vi "Wait.vi"(0 "Parallel Task in":refnum<k21>, 1 "PS type":enum16{"NHR", "ITECH"}(ring), 5 "P task error in":errorcluster, 9 "PS VISA in":refnum<visa-resource-name>, 11 "PS error in":errorcluster caption="NHR error in (no error)", 12 "Wait Filepath":path=path "C:/Users/ga11/Desktop/VI/results/3PtestChrgRest.lvm" caption="Filename", 13 "Wait time":dbl) -> (4 "parallel task out":refnum<k21>, 6 "parallel task error out":errorcluster, 10 "PS Visa Out":refnum<visa-resource-name>, 15 "PS error out":errorcluster)   [LabVIEW 2020]
uses:
  <instrlib>/NH Research Regenerative Test Series/Public/Data/Read (Ave Current).vi
  <instrlib>/NH Research Regenerative Test Series/Public/Data/Low Level/Fetch (Ave Voltage).vi
  <instrlib>/NH Research Regenerative Test Series/NH Research Regenerative Test Series.lvlib
  <instrlib>/IT-M3400/IT-M3400.lvlib
panel:
  out "Ave Current (A)":dbl
  out "Ave Voltage (V)":dbl
  out "WaitElapsed Time (s)":i32 caption="Elapsed Time (s)"
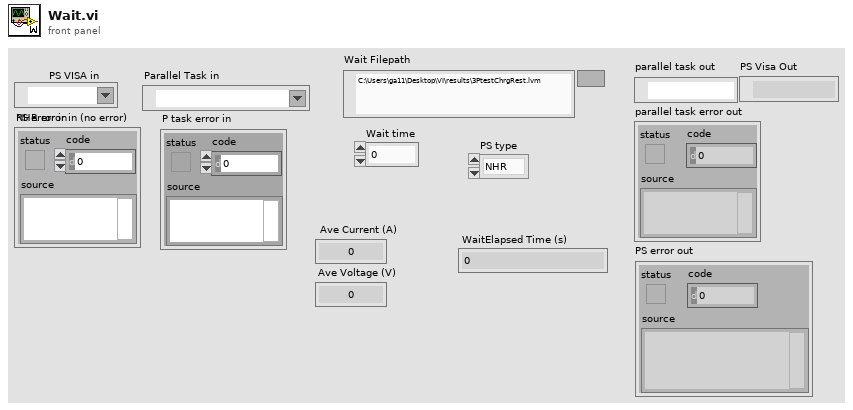
[diagram p1: front panel]
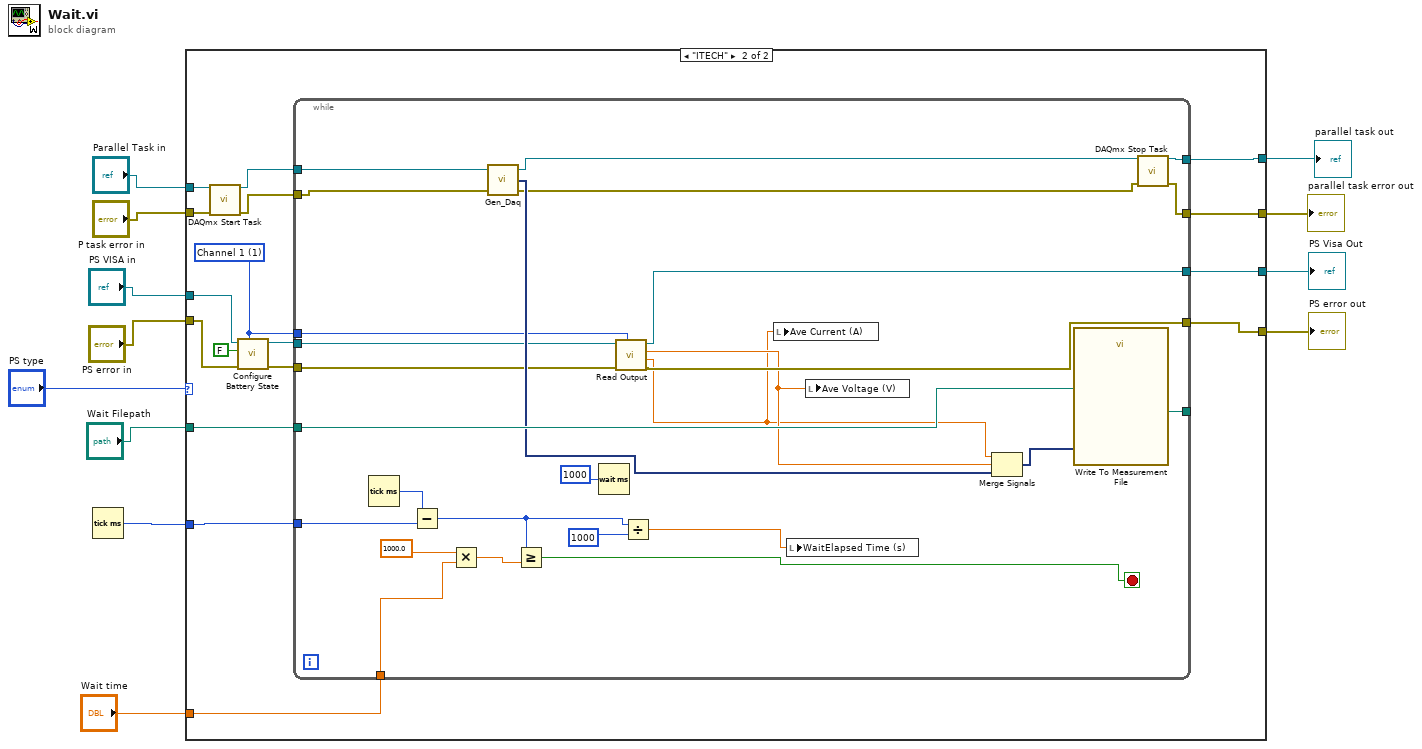
[diagram p0: block diagram]
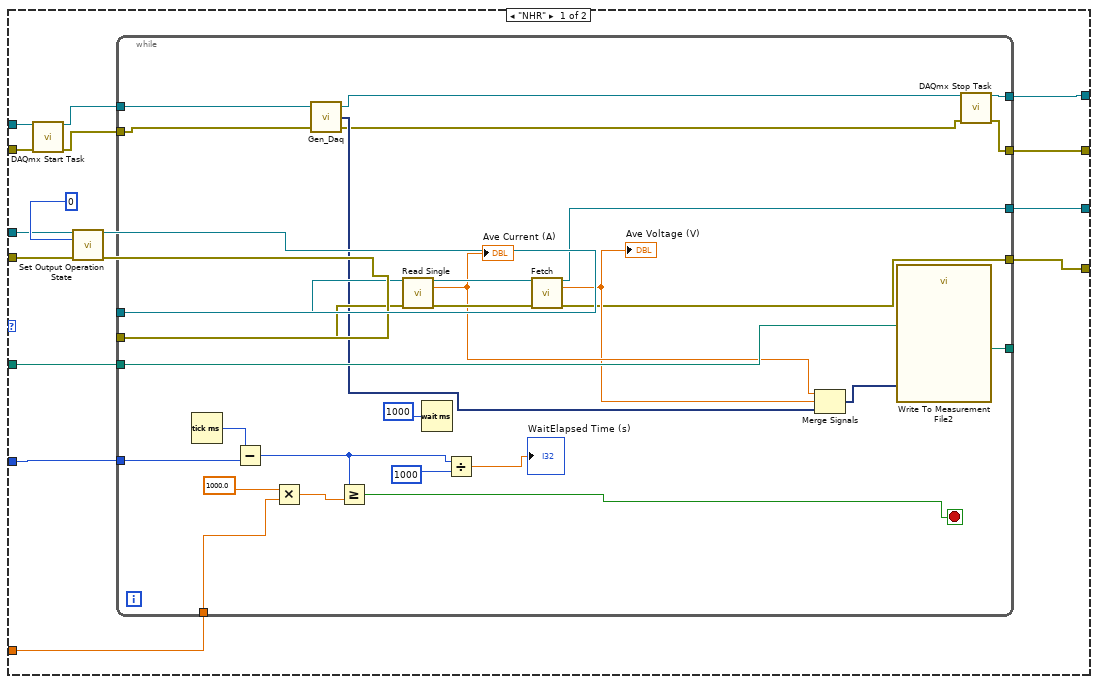
[diagram p2: hidden frame]
diagram:
  n1 = Tick Count (ms)() -> (millisecond timer value=w11:u32)
  n2 = case shown="\"ITECH\"" "PS type" {
    tunnel: "Wait time" -> [w25 w73]
    tunnel: w11 -> [w22 w70]
    tunnel: "Parallel Task in" -> [w21 w69]
    tunnel: "P task error in" -> [w20 w68]
    tunnel: "PS VISA in" -> [w19 w60]
    tunnel: "PS error in" -> [w18 w59]
    tunnel: "Wait Filepath" -> [w17 w67]
    tunnel: [w16 w66] -> w5
    tunnel: [w15 w65] -> w4
    tunnel: [w14 w64] -> w3
    tunnel: [w13 w63] -> w2
    frame "NHR" {
      n3 = call <vilib>:"DAQmx Start Task.vi"("task/channels in"=w21, "error in"=w20) -> ("task out"=w24:refnum<k21>, "error out"=w23:errorcluster)  [unwired: 12 in]
      n4 = call <vilib>:"Set Output Operation State.vi"("VISA resource name"=w19, "Mode (0: Off)"=0, "error in (no error)"=w18) -> ("VISA resource name out"=w27:refnum<visa-resource-name>, "error out"=w26:errorcluster)  [unwired: 11 in]
      n5 = while {
        tunnel: w27 -> [w54]
        tunnel: w26 -> [w53]
        tunnel: w25 -> [w49]
        tunnel: [w46] -> _
        tunnel: w24 -> [w36]
        tunnel: w23 -> [w35]
        tunnel: w22 -> [w45]
        tunnel: w17 -> [w44]
        tunnel: [w43] -> w16
        tunnel: [w42] -> w15
        tunnel: [w33] -> w14
        tunnel: [w32] -> w13
        stop <- w50 stop-if-true
        n6 = Tick Count (ms)() -> (millisecond timer value=w51:u32)
        n7 = Subtract(x=w51, y=w45) -> (x-y=w41:u32)
        n8 = Multiply(x=1000.0, y=w49) -> (x*y=w47:dbl)
        n9 = call "Gen_Daq.vi"("error in"=w35, "task/channels in"=w36) -> ("error out"=w29:errorcluster, "DaQ_output"=w31:dynamicdata, "task out"=w30:refnum<k21>)  [unwired: 1 in]
        n10 = Greater Or Equal?(x=w41, y=w47) -> (x >= y?=w50:bool)
        n11 = call-poly <instrlib>:"Read Single.vi"("VISA resource name"=w54, "error in (no error)"=w53) -> ("VISA resource name out"=w55:refnum<visa-resource-name>, "Ave Current (A)"=w38:dbl, "error out"=w56:errorcluster)  [unwired: 11 in]
        "Ave Current (A)" <- w38
        n12 = Wait (ms)(milliseconds to wait=1000) -> ()  [unwired: 1 out]
        n13 = Divide(x=w41, y=1000) -> (x/y=→"WaitElapsed Time (s)":dbl)
        n14 = call-poly <instrlib>:"Fetch.vi"("VISA resource name"=w55, "error in (no error)"=w56) -> ("VISA resource name out"=w33:refnum<visa-resource-name>, "Ave Voltage (V)"=w34:dbl, "error out"=w32:errorcluster)  [unwired: 11 in]
        "Ave Voltage (V)" <- w34
        n15 = Merge Signals "Merge Signals"(w38, w34, w31) -> (w37:dynamicdata)
        n16 = call "Write To Measurement File2"("Signals"=w37, "Filename"=w44) -> ("Filename Out"=w46:path)  [unwired: 15 in, 2 out]
        n17 = call <vilib>:"DAQmx Stop Task.vi"("task/channels in"=w30, "error in"=w29) -> ("task out"=w43:refnum<k21>, "error out"=w42:errorcluster)  [unwired: 12 in]
      }
    }
    frame "ITECH" {
      w57 = 1 items=["Channel 1"=1, "Channel 2"=2, "Channel 3"=3, "Channel 4"=4, "Channel 5"=5, "Channel 6"=6, "Channel 7"=7, "Channel 8"=8, "Channel 8"=9, "Channel 10"=10, "Channel 11"=11, "Channel 12"=12, "Channel 13"=13, "Channel 14"=14, "Channel 15"=15, "Channel 16"=16] ("Channel")
      n18 = call <vilib>:"DAQmx Start Task.vi"("task/channels in"=w69, "error in"=w68) -> ("task out"=w72:refnum<k21>, "error out"=w71:errorcluster)  [unwired: 12 in]
      n19 = call <instrlib>:"Configure Battery State.vi"("Channel"=w57, "error in"=w59, "State"=FALSE, "VISA resource name"=w60) -> ("error out"=w61:errorcluster, "VISA resource name out"=w62:refnum<visa-resource-name>)  [unwired: 6 in]
      n20 = while {
        tunnel: w73 -> [w97]
        tunnel: [w94] -> _
        tunnel: w72 -> [w86]
        tunnel: w71 -> [w85]
        tunnel: w70 -> [w93]
        tunnel: w67 -> [w92]
        tunnel: [w91] -> w66
        tunnel: [w90] -> w65
        tunnel: [w81] -> w64
        tunnel: [w80] -> w63
        tunnel: w62 -> [w76]
        tunnel: w61 -> [w75]
        tunnel: w57 -> [w74]
        stop <- w98 stop-if-true
        n21 = Tick Count (ms)() -> (millisecond timer value=w99:u32)
        n22 = Subtract(x=w99, y=w93) -> (x-y=w89:u32)
        n23 = Multiply(x=1000.0, y=w97) -> (x*y=w95:dbl)
        n24 = call "Gen_Daq.vi"("error in"=w85, "task/channels in"=w86) -> ("error out"=w82:errorcluster, "DaQ_output"=w84:dynamicdata, "task out"=w83:refnum<k21>)  [unwired: 1 in]
        n25 = Greater Or Equal?(x=w89, y=w95) -> (x >= y?=w98:bool)
        n26 = Wait (ms)(milliseconds to wait=1000) -> ()  [unwired: 1 out]
        n27 = call <instrlib>:"Read Output.vi"("Channel"=w74, "error in"=w75, "VISA resource name"=w76) -> ("error out"=w80:errorcluster, "Read Current(A)"=w78:dbl, "Read Voltage(V)"=w79:dbl, "VISA resource name out"=w81:refnum<visa-resource-name>)  [unwired: 5 in]
        n28 = Divide(x=w89, y=1000) -> (x/y=w77:dbl)
        n29 = local write "Ave Current (A)"(w78) -> ()
        n30 = local write "WaitElapsed Time (s)"(w77) -> ()
        n31 = local write "Ave Voltage (V)"(w79) -> ()
        n32 = Merge Signals "Merge Signals"(w78, w79, w84) -> (w87:dynamicdata)
        n33 = call "Write To Measurement File"("Signals"=w87, "Filename"=w92) -> ("Filename Out"=w94:path)  [unwired: 15 in, 2 out]
        n34 = call <vilib>:"DAQmx Stop Task.vi"("task/channels in"=w83, "error in"=w82) -> ("task out"=w91:refnum<k21>, "error out"=w90:errorcluster)  [unwired: 12 in]
      }
    }
  }
  "parallel task out" <- w5
  "parallel task error out" <- w4
  "PS Visa Out" <- w3
  "PS error out" <- w2
